vi "dfd_Read CFG File.vi"(8 "error in (no error)":errorcluster, 10 "section name":string, 11 "configuration file path":path) -> (0 "error out":errorcluster, 3 "Key Values":string[](array[string]))   [LabVIEW 2017, in "NI_DigFilterLicensed.lvlib"]
uses:
  <vilib>/addons/Digital Filter Design/NI_DigFilterLicensed.lvlib
  <vilib>/Utility/config.llb/Read Key (String).vi
  <vilib>/Utility/config.llb/NI_LVConfig.lvlib
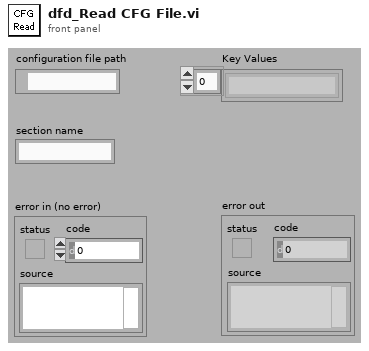
[diagram p1: front panel]
types:
  T1 = typedef "NI_LVConfig.lvlib/Config Data RefNum.ctl" = refnum<k1>
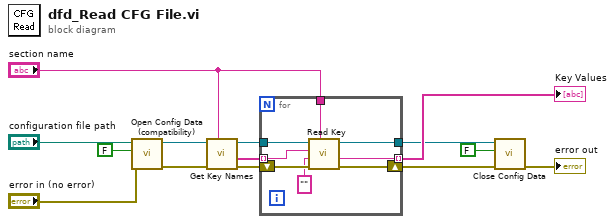
[diagram p0: block diagram]
diagram:
  n1 = call <vilib>:"Open Config Data (compatibility).vi"("error in (no error)"="error in (no error)", "create file if necessary (T)"=FALSE ("create file if necessary? (T)"), "configuration file path"="configuration file path") -> ("error out"=w11:errorcluster, "refnum"=w12:T1)  [unwired: 6 in, 1 out]
  n2 = call <vilib>:"Get Key Names.vi"("section"="section name", "error in (no error)"=w11, "refnum"=w12) -> ("error out"=w8:errorcluster, "key names"=w9:string[], "refnum out"=w10:T1)  [unwired: 6 out]
  n3 = for {
    tunnel: w10 -> [w22]
    tunnel: "section name" -> [w21]
    tunnel: w9 -> [w20] mode=indexing
    shift-right: [w18] -> w5
    shift-left: w8 -> [w19]
    tunnel: [w16] -> w6
    tunnel: [w15] -> w7 mode=indexing
    n4 = call-poly <vilib>:"Read Key.vi"("section"=w21, "error in (no error)"=w19, "default value"="", "key"=w20, "refnum"=w22) -> ("error out"=w18:errorcluster, "value"=w15:string, "refnum out"=w16:T1)  [unwired: 1 in, 3 out]
  }
  "Key Values" <- w7
  n5 = call <vilib>:"Close Config Data.vi"("error in (no error)"=w5, "write file if changed (T)"=FALSE ("write configuration file? (T)"), "refnum"=w6) -> ("error out"=→"error out":errorcluster)  [unwired: 8 out]
